vi "capstone1 ver 5.vi"() -> ()   [LabVIEW 2016]
uses:
  <instrlib>/Dynamixel Motor/Public/Motor Operation/Low Level/Baud Setting.ctl
  <vilib>/myRIO/Instrument Drivers/Onboard IO/DIO/typedefs/DIO Reference.ctl
  <vilib>/myRIO/Common/Instrument Driver Framework/Utilities/typedefs/myRIO Generic Hardware Reference.ctl
  <vilib>/myRIO/Common/Instrument Driver Framework/Utilities/typedefs/Hardware Version Enum.ctl
  <vilib>/myRIO/Common/Instrument Driver Framework/Utilities/typedefs/myRIO v1.0 Reference.ctl
  <vilib>/myRIO/Common/Instrument Driver Framework/Utilities/typedefs/Generic FPGA Reference.ctl
  <vilib>/myRIO/Common/Instrument Driver Framework/myRIO v1.0/DIO/typedefs/DIO Channels List.ctl
  <vilib>/myRIO/Common/Instrument Driver Framework/myRIO v1.0/DIO/typedefs/DIO Channels Enum.ctl
  <vilib>/userdefined/High Color/nirio_resource_hc.ctl
  <vilib>/myRIO/Common/Instrument Driver Framework/Utilities/vis/Is FPGA Ref Available.vi
  <vilib>/myRIO/Common/Instrument Driver Framework/myRIO v1.0/DIO/vis/myRIO v1.1 Open DIO.vi
  <vilib>/myRIO/Instrument Drivers/Onboard IO/DIO/vis/Write.vi
  <vilib>/myRIO/Common/Instrument Driver Framework/Utilities/vis/Validate Channels.vi
  <vilib>/myRIO/Common/Instrument Driver Framework/myRIO v1.0/DIO/vis/myRIO v1.0 Reserve DIO.vi
  <vilib>/myRIO/Common/Instrument Driver Framework/myRIO v1.0/UART/vis/myRIO v1.0 Close UART.vi
  <vilib>/myRIO/Common/Instrument Driver Framework/myRIO v1.0/Resource Manager/vis/myRIO v1.0 Reserve Channel List.vi
  <vilib>/myRIO/Common/Instrument Driver Framework/myRIO v1.0/DIO/vis/myRIO v1.0 Build MUX Configuration DIO.vi
  <vilib>/myRIO/Common/Instrument Driver Framework/myRIO v1.0/Resource Manager/vis/myRIO v1.0 Reserve Channel.vi
  <vilib>/myRIO/Common/Instrument Driver Framework/myRIO v1.0/Resource Manager/vis/myRIO v1.0 Unreserve Channel.vi
  <vilib>/myRIO/Common/Instrument Driver Framework/myRIO v1.0/Resource Manager/vis/myRIO v1.0 Create Configuration List.vi
  <vilib>/myRIO/Common/Instrument Driver Framework/myRIO v1.0/Resource Manager/vis/myRIO v1.0 Build Mutex Name.vi
  <vilib>/Utility/VariantDataType/GetNumericInfo.vi
  <vilib>/Utility/error.llb/Error Cluster From Error Code.vi
  <vilib>/myRIO/Common/Instrument Driver Framework/myRIO v1.0/myRIO v1.1 Open.vi
  <vilib>/myRIO/Common/Instrument Driver Framework/Utilities/vis/IO Manager.vi
  <vilib>/myRIO/Common/Instrument Driver Framework/Utilities/vis/Configuration Manager.vi
  <vilib>/myRIO/Common/Instrument Driver Framework/myRIO v1.0/Resource Manager/vis/myRIO v1.0 Configure IO.vi
  <vilib>/myRIO/Common/Instrument Driver Framework/myRIO v1.0/myRIO v1.0 Close.vi
  <vilib>/myRIO/Common/Instrument Driver Framework/myRIO v1.0/DIO/vis/myRIO v1.0 Write DIO.vi
  <vilib>/myRIO/Common/Instrument Driver Framework/Utilities/vis/FPGA Ref Manager.vi
  <vilib>/myRIO/Common/Instrument Driver Framework/myRIO v1.0/myRIO v1.0 Reset FPGA.vi
  <vilib>/myRIO/Common/Instrument Driver Framework/myRIO v1.0/IRQ/vis/myRIO v1.0 IRQ Info FGV.vi
  <vilib>/myRIO/Common/Instrument Driver Framework/myRIO v1.0/IRQ/vis/myRIO v1.0 Timer IRQ Info FGV.vi
  <vilib>/myRIO/Common/Instrument Driver Framework/myRIO v1.0/IRQ/vis/myRIO v1.0 ISR Agent.vi
  <vilib>/myRIO/Express VI/Onboard Devices/LED/LED Express VI.xnode
  <vilib>/myRIO/Instrument Drivers/Onboard IO/DIO/vis/myRIO DIO Open.xnode
  <instrlib>/Dynamixel Motor/Dynamixel Motor.lvlib
  <vilib>/myRIO/Instrument Drivers/Onboard IO/DIO/DIO.lvlib
  <vilib>/myRIO/Instrument Drivers/Utilities/Utilities.lvlib
panel:
  out "RT TCP Loop time 4":u32
  out "Numeric 2":i32
  out "RT TCP Loop time":u32
  out "motor temp":cluster{"0":sgl, "1":sgl, "2":sgl, "3":sgl}
  out "value":T1
  out "TCP Read data":string
  in  "정지":bool
  out "error out":errorcluster
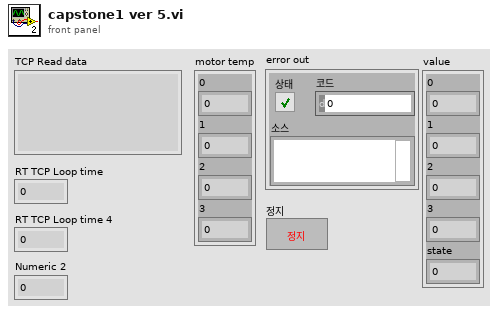
[diagram p1: front panel]
types:
  T1 = cluster{"0":sgl, "1":sgl, "2":sgl, "3":sgl, "state":sgl}
  T2 = typedef "Dynamixel Motor.lvlib/Baud Setting.ctl" = u8
  T3 = enum16{"big-endian, network order", "native, host order", "little-endian"}
  T4 = cluster{"0":sgl, "1":sgl, "2":sgl, "3":sgl, "state":i32}
  T5 = typedef "DIO.lvlib/DIO Reference.ctl" = cluster{"myRIO Reference":T6, "DIO Channels List":T10}
  T6 = typedef "myRIO Generic Hardware Reference.ctl" = cluster{"myRIO Model":T7, "myRIO Hardware Reference":T8}
  T7 = typedef "Hardware Version Enum.ctl" = enum16{"Unknown", "myRIO-1900", "myRIO-1950", "roboRIO", "NI ELVIS RIO CM"}
  T8 = typedef "myRIO v1.0 Reference.ctl" = cluster{"Generic FPGA Reference":T9, "Allow multiple opens":bool}
  T9 = typedef "Generic FPGA Reference.ctl" = refnum<k20>
  T10 = typedef "DIO Channels List.ctl" = T11[]
  T11 = typedef "DIO Channels Enum.ctl" = enum16{"Not Connected", "C/DIO0", "C/DIO1", "C/DIO2", "C/DIO3", "C/DIO4", "C/DIO5", "C/DIO6", "C/DIO7", "A/DIO0", "A/DIO1", "A/DIO2", "A/DIO3", "A/DIO4", "A/DIO5", "A/DIO6", "A/DIO7", "A/DIO8", "A/DIO9", "A/DIO10", "A/DIO11", "A/DIO12", "A/DIO13", "A/DIO14", "A/DIO15", "B/DIO0", "B/DIO1", "B/DIO2", "B/DIO3", "B/DIO4", "B/DIO5", "B/DIO6", "B/DIO7", "B/DIO8", "B/DIO9", "B/DIO10", "B/DIO11", "B/DIO12", "B/DIO13", "B/DIO14", "B/DIO15", "LED0", "LED1", "LED2", "LED3", "Button0", "DIO/DIO0", "DIO/DIO1", "DIO/DIO2", "DIO/DIO3", "DIO/DIO4", "DIO/DIO5", "DIO/DIO6", "DIO/DIO7", "DIO/DIO8", "DIO/DIO9", "SPI/CS0", "SPI/CS1", "SPI/CS2", "SPI/CS3", "LED RADIO (Green)", "LED RADIO (Red)", "LED COMM (Green)", "LED COMM (Red)", "LED MODE (Green)", "LED MODE (Red)"}
  T12 = typedef "nirio_resource_hc.ctl" = tag
  T13 = cluster{"Temperature (C)":u8, "Temperature (C)":u8, "Temperature (C)":u8, "Temperature (C)":u8}
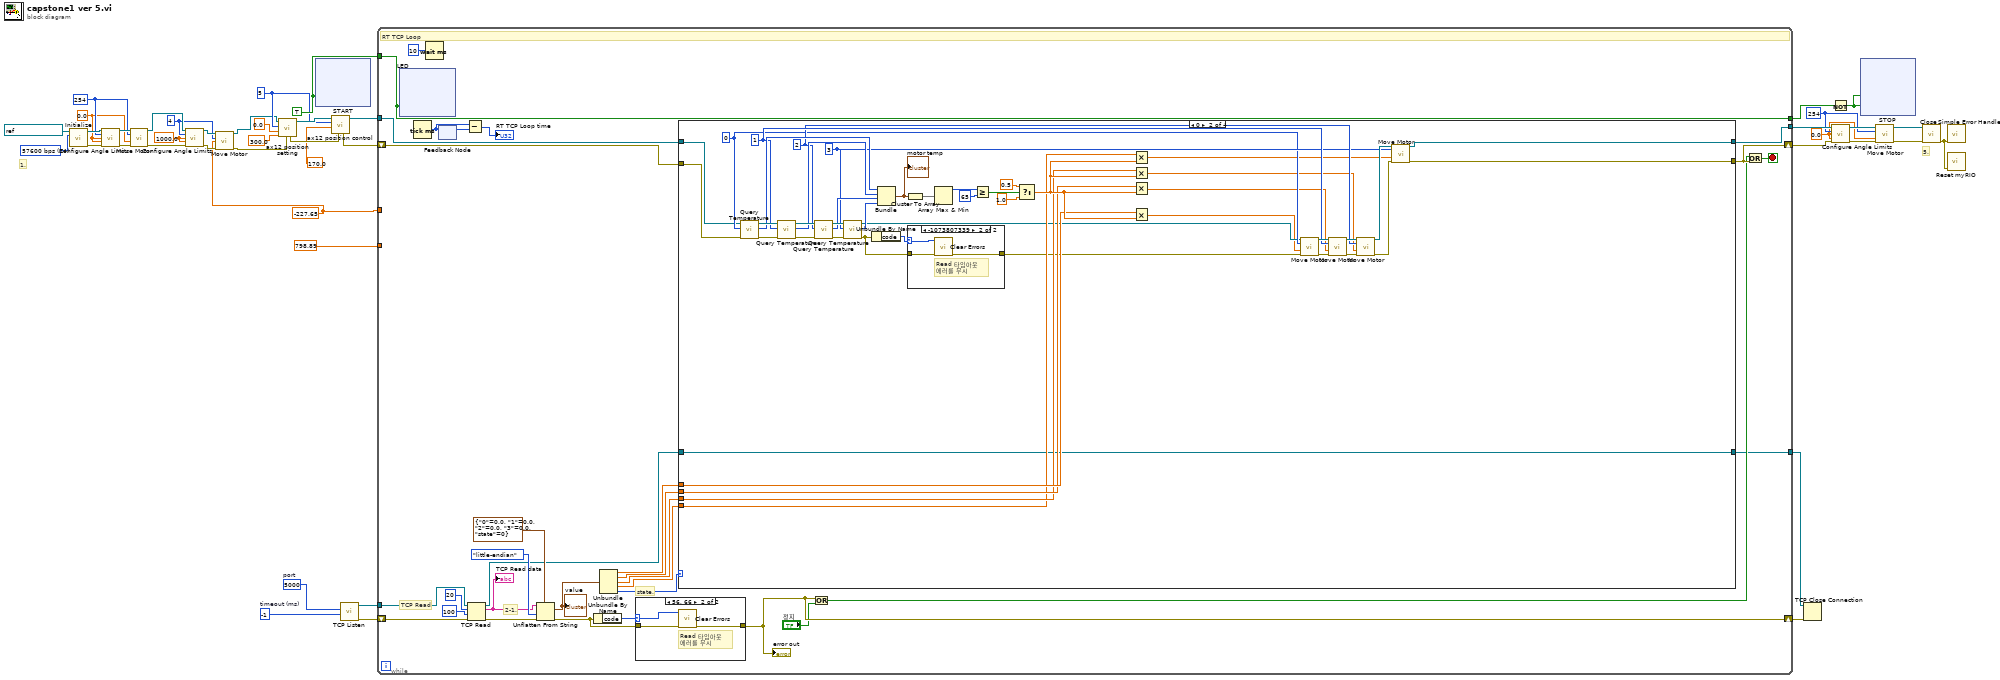
[diagram p0: block diagram]
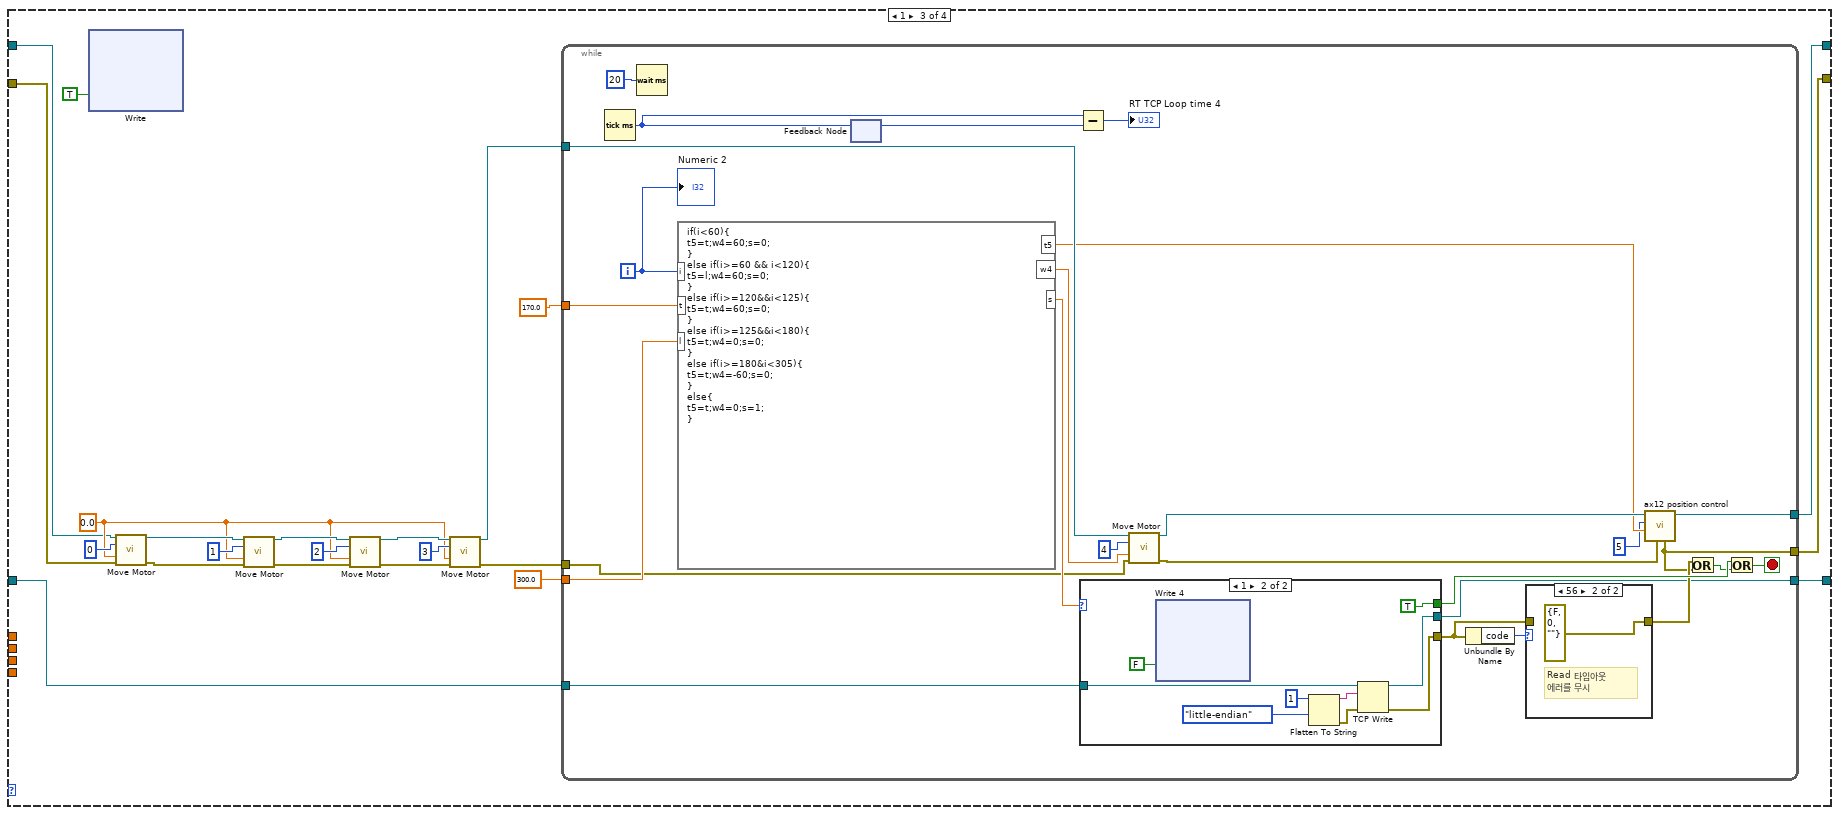
[diagram p4: hidden frame]
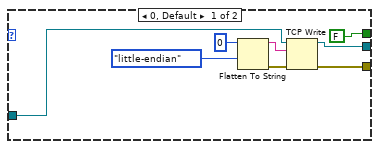
[diagram p6: hidden frame]
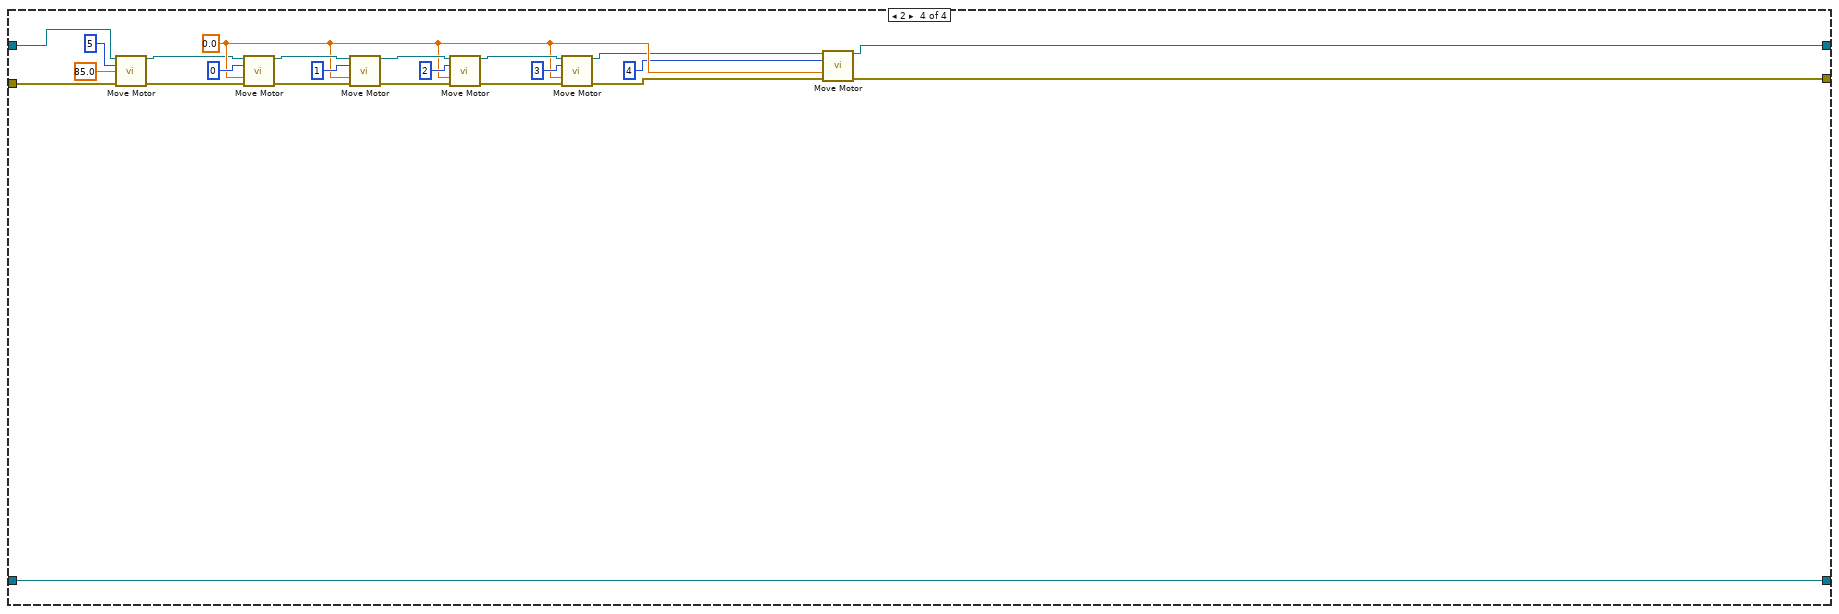
[diagram p7: hidden frame]
diagram:
  w2 = -227.65 ("Goal Position (180 deg)")
  w22 = 1000.0 ("Clockwise Angle Limit (0 deg)")
  w3 = 4
  w14 = 5
  w39 = T2 34 items=["1,000,000 bps"=1, "500,000 bps"=3, "400,000 bps"=4, "250,000 bps"=7, "200,000 bps"=9, "115200 bps"=16, "57600 bps"=34, "19200 bps"=103, "9600 bps"=207] ("Baud rate (57600 bps)")
  w29 = TRUE
  w8 = 0.0 ("Goal Speed (RPM)")
  w9 = u8 254 ("Motor ID (0)")
  w31 = u8 254 ("Motor ID (0)")
  w30 = 0.0 ("Clockwise Angle Limit (0 deg)")
  w43 = u16 5000  # port
  w44 = -1  # timeout (ms)
  # "5."
  # "1."
  n1 = call <instrlib>:"Initialize.vi"("Baud rate (57600 bps)"=w39, "VISA resource name"=refnum<visa-resource-name> "ASRL3::INSTR") -> ("error out"=w35:errorcluster, "VISA resource name out"=w34:refnum<visa-resource-name>)  [unwired: 8 in]
  n2 = call <instrlib>:"Configure Angle Limits.vi"("VISA resource name"=w34, "Motor ID (0)"=w31, "Clockwise Angle Limit (0 deg)"=w30, "Counter-Clockwise Angle Limit (300 deg)"=w30, "error in (no error)"=w35) -> ("VISA resource name out"=w33:refnum<visa-resource-name>, "error out"=w32:errorcluster)  [unwired: 9 in]
  n3 = call <instrlib>:"Move Motor.vi"("VISA resource name"=w33, "Motor ID (0)"=w31, "Goal Speed (RPM)"=w30, "error in (no error)"=w32) -> ("VISA resource name out"=w24:refnum<visa-resource-name>, "error out"=w23:errorcluster)  [unwired: 10 in]
  n4 = call <instrlib>:"Configure Angle Limits.vi"("VISA resource name"=w24, "Motor ID (0)"=w3, "Clockwise Angle Limit (0 deg)"=w22, "Counter-Clockwise Angle Limit (300 deg)"=w22, "error in (no error)"=w23) -> ("VISA resource name out"=w7:refnum<visa-resource-name>, "error out"=w4:errorcluster)  [unwired: 9 in]
  n5 = call <instrlib>:"Move Motor.vi"("VISA resource name"=w7, "Motor ID (0)"=w3, "Goal Position (180 deg)"=w2, "error in (no error)"=w4) -> ("VISA resource name out"=w6:refnum<visa-resource-name>, "error out"=w5:errorcluster)  [unwired: 10 in]
  n6 = call "ax12 position setting.vi"("error in (no error)"=w5, "Counter-Clockwise Angle Limit (300 deg)"=300.0 ("Clockwise Angle Limit (0 deg)"), "Clockwise Angle Limit (0 deg)"=0.0, "Motor ID (0)"=w14, "VISA resource name"=w6) -> ("VISA resource name out"=w19:refnum<visa-resource-name>, "error out"=w16:errorcluster)  [unwired: 5 in]
  n7 = xnode "START"("LED0"=w29) -> ()  [unwired: 1 in, 1 out]
  n8 = call "ax12 position control.vi"("error in (no error)"=w16, "Goal Position (180 deg)"=170.0, "Motor ID (0)"=w14, "VISA resource name"=w19) -> ("VISA resource name out"=w18:refnum<visa-resource-name>, "error out"=w17:errorcluster)  [unwired: 6 in]
  n9 = call <vilib>:"TCP Listen.vi"("timeout ms (wait forever: -1)"=w44, "port"=w43) -> ("error out"=w40:errorcluster, "connection ID"=w26:refnum<k5>)  [unwired: 5 in, 3 out]
  n10 = while {
    tunnel: w26 -> [w65]
    tunnel: [w45] -> w42
    shift-right: [w50] -> w41
    shift-left: w40 -> [w66]
    shift-right: [w56] -> w13
    shift-left: w17 -> [w55]
    tunnel: w29 -> [w64]
    tunnel: [w64] -> w37
    tunnel: [w57] -> w11
    tunnel: w18 -> [w47]
    tunnel: w2 -> [_]
    tunnel: 798.89 ("Goal Position (180 deg)") -> [_]
    stop <- w48 stop-if-true
    # "state."
    # "2-1."
    # "TCP Read"
    # "RT TCP Loop"
    n11 = xnode "LED"("LED1"=w64) -> ()  [unwired: 1 in, 1 out]
    n12 = Tick Count (ms)() -> (millisecond timer value=w52:u32)
    n13 = Wait (ms)(milliseconds to wait=u32 10 ("대기 시간 (ms)")) -> ()  [unwired: 1 out]
    n14 = feedback #1() -> (w53:u32)  [unwired: 1 in]
    n15 = feedback-in #1(w52) -> ()
    n16 = Subtract(x=w52, y=w53) -> (x-y=→"RT TCP Loop time":u32)
    n17 = TCP Read(connection ID=w65, bytes to read=20 ("읽을 바이트"), error in (no error)=w66, 9:100 ("타임아웃 ms (25000)")) -> (connection ID out=w46:refnum<k5>, data out=w69:string, error out=w68:errorcluster)  [unwired: 1 in]
    "TCP Read data" <- w69
    n18 = Unflatten From String(type=T4 {"0"=0.0, "1"=0.0, "2"=0.0, "3"=0.0, "state"=0}, binary string=w69, byte order (0:big-endian, network order)=T3."little-endian", error in (no error)=w68) -> (value=w63:T4, error out=w67:errorcluster)  [unwired: 1 in, 1 out]
    "value" <- w63
    n19 = Unbundle By Name(w67) -> ("code"=w74:i32)
    n20 = Unbundle(w63) -> ("0"=w62:sgl, "1"=w60:sgl, "2"=w61:sgl, "3"=w59:sgl, "state"=w58:i32)
    n21 = case shown="56, 66" w74 {
      selector: w74 -> [_ w325]
      tunnel: [w323 w324] -> w50
      tunnel: w67 -> [w323 w326]
      frame 0, Default {
      }
      frame 56, 66 {
        # "Read 타임아웃\n에러를 무시"
        n22 = call <vilib>:"Clear Errors.vi"("error in (no error)"=w326, "specific error code to clear (0: all)"=w325) -> ("error out"=w324:errorcluster)  [unwired: 4 in, 1 out]
      }
    }
    "error out" <- w50
    n23 = case shown="0" w58 {
      tunnel: w62 -> [_ w107 _ _]
      tunnel: w60 -> [_ w106 _ _]
      tunnel: w61 -> [_ w105 _ _]
      tunnel: w59 -> [_ w104 _ _]
      tunnel: [w78 w89 w132 w274] -> w57
      tunnel: [w77 w90 w128 w273] -> w56
      tunnel: w55 -> [w77 w87 w138 w270]
      tunnel: w47 -> [w78 w80 w136 w266]
      tunnel: w46 -> [w76 w79 w131 w265]
      tunnel: [w76 w79 w130 w265] -> w45
      frame -1, Default {
      }
      frame 0 {
        w91 = 3
        w92 = 2
        w93 = 1
        w88 = 0
        n24 = call <instrlib>:"Query Temperature.vi"("error in"=w87, "Motor ID (0)"=w88, "VISA resource name"=w80) -> ("error out"=w114:errorcluster, "Temperature (C)"=w103:u8, "VISA resource name out"=w117:refnum<visa-resource-name>)  [unwired: 6 in]
        n25 = call <instrlib>:"Query Temperature.vi"("error in"=w114, "Motor ID (0)"=w93, "VISA resource name"=w117) -> ("error out"=w113:errorcluster, "Temperature (C)"=w102:u8, "VISA resource name out"=w116:refnum<visa-resource-name>)  [unwired: 6 in]
        n26 = call <instrlib>:"Query Temperature.vi"("error in"=w113, "Motor ID (0)"=w92, "VISA resource name"=w116) -> ("error out"=w112:errorcluster, "Temperature (C)"=w101:u8, "VISA resource name out"=w115:refnum<visa-resource-name>)  [unwired: 6 in]
        n27 = call <instrlib>:"Query Temperature.vi"("error in"=w112, "Motor ID (0)"=w91, "VISA resource name"=w115) -> ("error out"=w94:errorcluster, "Temperature (C)"=w100:u8, "VISA resource name out"=w86:refnum<visa-resource-name>)  [unwired: 6 in]
        n28 = Unbundle By Name(w94) -> ("code"=w95:i32)
        n29 = Bundle("Temperature (C)"=w103, "Temperature (C)"=w102, "Temperature (C)"=w101, "Temperature (C)"=w100) -> (w97:T13)  [unwired: 1 in]
        "motor temp" <- w97
        n30 = Cluster To Array(cluster=w97) -> (array=w99:u8[])
        n31 = case shown="-1073807339" w95 {
          selector: w95 -> [_ w126]
          tunnel: [w124 w125] -> w85
          tunnel: w94 -> [w124 w127]
          frame 0, Default {
          }
          frame -1073807339 {
            # "Read 타임아웃\n에러를 무시"
            n32 = call <vilib>:"Clear Errors.vi"("error in (no error)"=w127, "specific error code to clear (0: all)"=w126) -> ("error out"=w125:errorcluster)  [unwired: 4 in, 1 out]
          }
        }
        n33 = Array Max & Min(array=w99) -> (max value=w98:u8)  [unwired: 3 out]
        n34 = Greater Or Equal?(x=w98, y=65) -> (x >= y?=w96:bool)
        n35 = Select(t=0.5, s=w96, f=1.0) -> (s? t:f=w108:dbl)
        n36 = Multiply(x=w104, y=w108) -> (x*y=w81:dbl)
        n37 = Multiply(x=w105, y=w108) -> (x*y=w82:dbl)
        n38 = Multiply(x=w106, y=w108) -> (x*y=w83:dbl)
        n39 = Multiply(x=w107, y=w108) -> (x*y=w84:dbl)
        n40 = call <instrlib>:"Move Motor.vi"("VISA resource name"=w86, "Motor ID (0)"=w88, "Goal Speed (RPM)"=w84, "error in (no error)"=w85) -> ("VISA resource name out"=w118:refnum<visa-resource-name>, "error out"=w119:errorcluster)  [unwired: 10 in]
        n41 = call <instrlib>:"Move Motor.vi"("VISA resource name"=w118, "Motor ID (0)"=w93, "Goal Speed (RPM)"=w83, "error in (no error)"=w119) -> ("VISA resource name out"=w120:refnum<visa-resource-name>, "error out"=w122:errorcluster)  [unwired: 10 in]
        n42 = call <instrlib>:"Move Motor.vi"("VISA resource name"=w120, "Motor ID (0)"=w92, "Goal Speed (RPM)"=w82, "error in (no error)"=w122) -> ("VISA resource name out"=w121:refnum<visa-resource-name>, "error out"=w123:errorcluster)  [unwired: 10 in]
        n43 = call <instrlib>:"Move Motor.vi"("VISA resource name"=w121, "Motor ID (0)"=w91, "Goal Speed (RPM)"=w81, "error in (no error)"=w123) -> ("VISA resource name out"=w89:refnum<visa-resource-name>, "error out"=w90:errorcluster)  [unwired: 10 in]
      }
      frame 1 {
        w139 = 0.0
        n44 = xnode "Write"("LED2"=TRUE) -> ()  [unwired: 1 in, 1 out]
        n45 = call <instrlib>:"Move Motor.vi"("VISA resource name"=w136, "Motor ID (0)"=0, "Goal Speed (RPM)"=w139, "error in (no error)"=w138) -> ("VISA resource name out"=w140:refnum<visa-resource-name>, "error out"=w141:errorcluster)  [unwired: 10 in]
        n46 = call <instrlib>:"Move Motor.vi"("VISA resource name"=w140, "Motor ID (0)"=1, "Goal Speed (RPM)"=w139, "error in (no error)"=w141) -> ("VISA resource name out"=w142:refnum<visa-resource-name>, "error out"=w144:errorcluster)  [unwired: 10 in]
        n47 = call <instrlib>:"Move Motor.vi"("VISA resource name"=w142, "Motor ID (0)"=2, "Goal Speed (RPM)"=w139, "error in (no error)"=w144) -> ("VISA resource name out"=w143:refnum<visa-resource-name>, "error out"=w145:errorcluster)  [unwired: 10 in]
        n48 = call <instrlib>:"Move Motor.vi"("VISA resource name"=w143, "Motor ID (0)"=3, "Goal Speed (RPM)"=w139, "error in (no error)"=w145) -> ("VISA resource name out"=w133:refnum<visa-resource-name>, "error out"=w129:errorcluster)  [unwired: 10 in]
        n49 = while {
          tunnel: w131 -> [w171]
          tunnel: w133 -> [w175]
          tunnel: [w154] -> w132
          tunnel: 170.0 -> [w170]
          tunnel: 300.0 -> [w169]
          tunnel: [w152] -> w128
          tunnel: [w157] -> w130
          tunnel: w129 -> [w156]
          i -> [w173]
          stop <- w160 stop-if-true
          n50 = Tick Count (ms)() -> (millisecond timer value=w166:u32)
          n51 = Wait (ms)(milliseconds to wait=u32 20 ("대기 시간 (ms)")) -> ()  [unwired: 1 out]
          n52 = formula code="if(i<60){\nt5=t;w4=60;s=0;\n}\nelse if(i>=60 && i<120){\nt5=l;w4=60;s=0;\n}\nelse if(i>=120&&i<125){\nt5=t;w4=60;s=0;\n}\nelse if(i>=125&&i<180){\nt5=t;w4=0;s=0;\n}\nelse if(i>=180&i<305){\nt5=t;w4=-60;s=0;\n}\nelse{\nt5=t;w4=0;s=1;\n}"("i"=w173, "t"=w170, "l"=w169) -> ("t5"=w151:dbl, "w4"=w172:dbl, "s"=w168:dbl)
          n53 = feedback #2() -> (w167:u32)  [unwired: 1 in]
          n54 = feedback-in #2(w166) -> ()
          n55 = Subtract(x=w166, y=w167) -> (x-y=→"RT TCP Loop time 4":u32)
          n56 = case shown="1" w168 {
            tunnel: w171 -> [w182 w194]
            tunnel: [FALSE TRUE] -> w164
            tunnel: [w179 w188] -> w162
            tunnel: [w178 w186] -> w157
            frame 0, Default {
              n57 = Flatten To String(anything=0, byte order (0:big-endian, network order)=T3."little-endian") -> (data string=w183:string, error out=w180:errorcluster)  [unwired: 2 in, 1 out]
              n58 = TCP Write(connection ID=w182, data in=w183, error in (no error)=w180) -> (connection ID out=w178:refnum<k5>, error out=w179:errorcluster)  [unwired: 1 in, 1 out]
            }
            frame 1 {
              n59 = xnode "Write 4"("LED2"=FALSE ("notification")) -> ()  [unwired: 1 in, 1 out]
              n60 = Flatten To String(anything=1, byte order (0:big-endian, network order)=T3."little-endian") -> (data string=w191:string, error out=w189:errorcluster)  [unwired: 2 in, 1 out]
              n61 = TCP Write(connection ID=w194, data in=w191, error in (no error)=w189) -> (connection ID out=w186:refnum<k5>, error out=w188:errorcluster)  [unwired: 1 in, 1 out]
            }
          }
          n62 = call <instrlib>:"Move Motor.vi"("VISA resource name"=w175, "Motor ID (0)"=4, "Goal Speed (RPM)"=w172, "error in (no error)"=w156) -> ("VISA resource name out"=w155:refnum<visa-resource-name>, "error out"=w153:errorcluster)  [unwired: 10 in]
          n63 = Unbundle By Name(w162) -> ("code"=w163:i32)
          n64 = case shown="56" w163 {
            tunnel: [w176 errorcluster {"status"=FALSE, "code"=0, "source"=""} ("에러 출력")] -> w161
            tunnel: w162 -> [w176 _]
            frame 0, Default {
            }
            frame 56 {
              # "Read 타임아웃\n에러를 무시"
            }
          }
          n65 = call "ax12 position control.vi"("error in (no error)"=w153, "Goal Position (180 deg)"=w151, "Motor ID (0)"=5, "VISA resource name"=w155) -> ("VISA resource name out"=w154:refnum<visa-resource-name>, "error out"=w152:errorcluster)  [unwired: 6 in]
          n66 = Or(x=w161, y=w152) -> (x .or. y?=w158:bool)
          n67 = Or(x=w164, y=w158) -> (x .or. y?=w160:bool)
          "Numeric 2" <- w173
        }
      }
      frame 2 {
        w277 = 0.0
        n68 = call <instrlib>:"Move Motor.vi"("VISA resource name"=w266, "Motor ID (0)"=5, "Goal Position (180 deg)"=85.0, "error in (no error)"=w270) -> ("VISA resource name out"=w268:refnum<visa-resource-name>, "error out"=w269:errorcluster)  [unwired: 10 in]
        n69 = call <instrlib>:"Move Motor.vi"("VISA resource name"=w268, "Motor ID (0)"=0, "Goal Speed (RPM)"=w277, "error in (no error)"=w269) -> ("VISA resource name out"=w287:refnum<visa-resource-name>, "error out"=w286:errorcluster)  [unwired: 10 in]
        n70 = call <instrlib>:"Move Motor.vi"("VISA resource name"=w287, "Motor ID (0)"=1, "Goal Speed (RPM)"=w277, "error in (no error)"=w286) -> ("VISA resource name out"=w285:refnum<visa-resource-name>, "error out"=w283:errorcluster)  [unwired: 10 in]
        n71 = call <instrlib>:"Move Motor.vi"("VISA resource name"=w285, "Motor ID (0)"=2, "Goal Speed (RPM)"=w277, "error in (no error)"=w283) -> ("VISA resource name out"=w284:refnum<visa-resource-name>, "error out"=w282:errorcluster)  [unwired: 10 in]
        n72 = call <instrlib>:"Move Motor.vi"("VISA resource name"=w284, "Motor ID (0)"=3, "Goal Speed (RPM)"=w277, "error in (no error)"=w282) -> ("VISA resource name out"=w275:refnum<visa-resource-name>, "error out"=w272:errorcluster)  [unwired: 10 in]
        n73 = call <instrlib>:"Move Motor.vi"("VISA resource name"=w275, "Motor ID (0)"=4, "Goal Speed (RPM)"=w277, "error in (no error)"=w272) -> ("VISA resource name out"=w274:refnum<visa-resource-name>, "error out"=w273:errorcluster)  [unwired: 10 in]
      }
    }
    n74 = Or(x=w50, y="정지") -> (x .or. y?=w54:bool)
    n75 = Or(x=w54, y=w56) -> (x .or. y?=w48:bool)
  }
  n76 = TCP Close Connection(connection ID=w42, error in (no error)=w41) -> ()  [unwired: 3 out]
  n77 = Not(x=w37) -> (.not. x?=w36:bool)
  n78 = call <instrlib>:"Configure Angle Limits.vi"("VISA resource name"=w11, "Motor ID (0)"=w9, "Clockwise Angle Limit (0 deg)"=w8, "Counter-Clockwise Angle Limit (300 deg)"=w8, "error in (no error)"=w13) -> ("VISA resource name out"=w10:refnum<visa-resource-name>, "error out"=w12:errorcluster)  [unwired: 9 in]
  n79 = xnode "STOP"("LED0"=w36, "LED1"=w36) -> ()  [unwired: 1 in, 1 out]
  n80 = call <instrlib>:"Move Motor.vi"("VISA resource name"=w10, "Motor ID (0)"=w9, "Goal Speed (RPM)"=w8, "error in (no error)"=w12) -> ("VISA resource name out"=w28:refnum<visa-resource-name>, "error out"=w27:errorcluster)  [unwired: 10 in]
  n81 = call <instrlib>:"Close.vi"("error in (no error)"=w27, "VISA resource name"=w28) -> ("error out"=w25:errorcluster)  [unwired: 9 in]
  n82 = call <vilib>:"Simple Error Handler.vi"("error in (no error)"=w25) -> ()  [unwired: 4 in, 5 out]
  n83 = call <vilib>:"Reset myRIO.vi"("error in (no error)"=w25) -> ()  [unwired: 10 in, 1 out]
